vi "Station Parse Instrument Info Only.vi"(8 "error in (no error)":errorcluster, 11 "Station in":refnum<class "Station.lvclass">) -> (0 "error out":errorcluster, 2 "Inst Info only output":string[][](array[string]), 3 "Station out":refnum<class "Station.lvclass">)   [LabVIEW 2018, in "Station.lvclass"]
uses:
  Station.lvclass
  Station.lvclass/Station.ctl
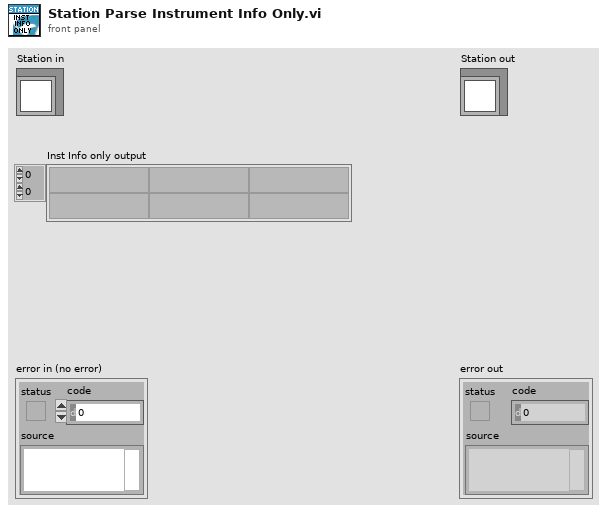
[diagram p1: front panel]
types:
  T1 = typedef "Station Initialize Data.ctl" = string[][]
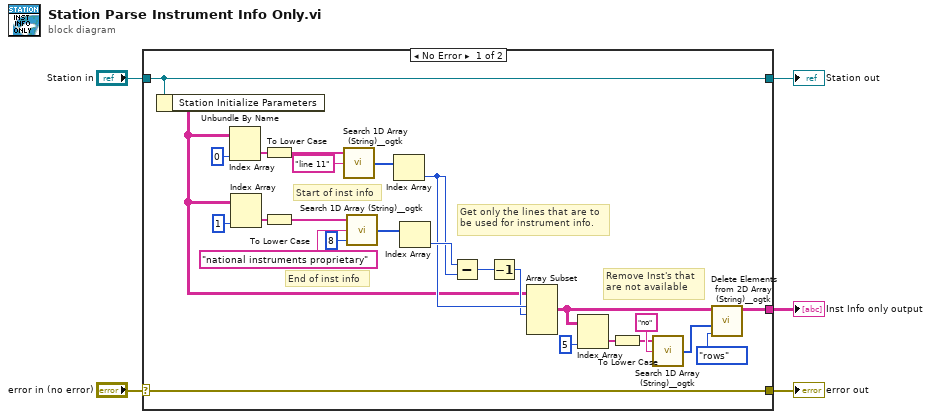
[diagram p0: block diagram]
diagram:
  n1 = case shown="No Error" "error in (no error)" {
    selector: "error in (no error)" -> [w18 w33]
    tunnel: [w18 w33] -> w3
    tunnel: [w10 _] -> w5
    tunnel: "Station in" -> [w7 w32]
    tunnel: [w7 w32] -> w1
    frame No Error {
      # "Remove Inst's that\nare not available"
      # "Get only the lines that are to\nbe used for instrument info."
      # "End of inst info"
      # "Start of inst info"
      n2 = Unbundle By Name(w7) -> ("Station Initialize Parameters"=w6:T1)
      n3 = Index Array(array=w6, index (col)=0 ("disabled index (col)")) -> (element=w19:string[])  [unwired: 1 in]
      n4 = Index Array(array=w6, index (col)=1 ("disabled index (col)")) -> (element=w20:string[])  [unwired: 1 in]
      n5 = To Lower Case(string=w19) -> (all lower case string=w17:string[])
      n6 = To Lower Case(string=w20) -> (all lower case string=w16:string[])
      n7 = call <userlib>:"Search 1D Array (String)__ogtk.vi"("Array"=w17, "Element Data"="line 11") -> ("Indices of Elements"=w27:i32[])  [unwired: 7 in]
      n8 = call <userlib>:"Search 1D Array (String)__ogtk.vi"("Array"=w16, "Element Data"="national instruments proprietary", "Start Index (0)"=8) -> ("Indices of Elements"=w26:i32[])  [unwired: 6 in]
      n9 = Index Array(array=w27) -> (element=w23:i32)  [unwired: 1 in]
      n10 = Index Array(array=w26) -> (element=w24:i32)  [unwired: 1 in]
      n11 = Subtract(x=w24, y=w23) -> (x-y=w22:i32)
      n12 = Decrement(x=w22) -> (x-1=w21:i32)
      n13 = Array Subset(array=w6, index (row)=w23, length (row)=w21) -> (w11:T1)  [unwired: 2 in]
      n14 = Index Array(array=w11, index (col)=5 ("disabled index (col)")) -> (element=w14:string[])  [unwired: 1 in]
      n15 = To Lower Case(string=w14) -> (all lower case string=w12:string[])
      n16 = call <userlib>:"Search 1D Array (String)__ogtk.vi"("Array"=w12, "Element Data"="no") -> ("Indices of Elements"=w9:i32[])  [unwired: 7 in]
      n17 = call <userlib>:"Delete Elements from 2D Array (String)__ogtk.vi"("delete (rows or columns)"=enum16{"rows", "columns"}."rows", "indices"=w9, "array"=w11) -> ("array w/ subset deleted"=w10:string[][])  [unwired: 7 in, 1 out]
    }
    frame Error {
    }
  }
  "error out" <- w3
  "Station out" <- w1
  "Inst Info only output" <- w5
